vi "roboRIO v1.0 Enable Encoder.vi"(8 "error in (no error)":errorcluster, 9 "Enable":bool, 10 "Channel":T1, 11 "myRIO Ref In":T2) -> (0 "error out":errorcluster, 3 "myRIO Ref Out":T2)   [LabVIEW 2021]
uses:
  <vilib>/myRIO/Common/Instrument Driver Framework/Utilities/typedefs/myRIO v1.0 Reference.ctl
  <vilib>/myRIO/Common/Instrument Driver Framework/Utilities/typedefs/Generic FPGA Reference.ctl
  <vilib>/myRIO/Common/Instrument Driver Framework/myRIO v1.0/Encoder/typedefs/Encoder Channels Enum.ctl
  <vilib>/myRIO/Common/Instrument Driver Framework/roboRIO v1.0/Encoder/typedefs/roboRIO Encoder Channels FPGA Reference.ctl
  <vilib>/rvi/errors/niLvFpgaAdjustHostInterfaceError.vi
  <vilib>/rvi/interface/nirviReadWriteControl/nirviReadWriteControl.xnode
  <vilib>/rvi/interface/Simulation/niFpgaSimulationCallBeginRW.vi
  NiFpgaLv.dll
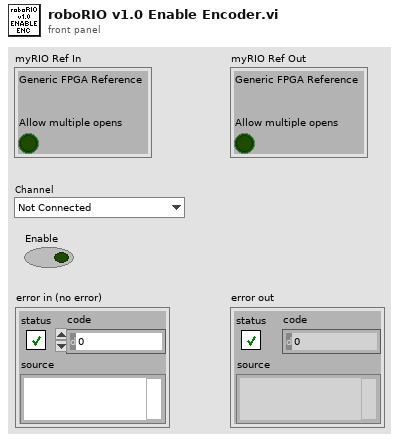
[diagram p1: front panel]
types:
  T1 = typedef "Encoder Channels Enum.ctl" = enum16{"Not Connected", "C/ENC0", "C/ENC1", "A/ENC", "A/ENC0", "A/ENC1", "A/ENC2", "A/ENC3", "A/ENC4", "A/ENC5", "A/ENC6", "A/ENC7", "A/ENC8", "A/ENC9", "B/ENC", "B/ENC0", "B/ENC1", "B/ENC2", "B/ENC3", "B/ENC4", "B/ENC5", "B/ENC6", "B/ENC7", "B/ENC8", "B/ENC9", "DIO/ENC0", "DIO/ENC1", "DIO/ENC2", "DIO/ENC3", "DIO/ENC4"}
  T2 = typedef "myRIO v1.0 Reference.ctl" = cluster{"Generic FPGA Reference":T3, "Allow multiple opens":bool}
  T3 = typedef "Generic FPGA Reference.ctl" = refnum<k20>
  T4 = typedef "roboRIO Encoder Channels FPGA Reference.ctl" = refnum<k20>
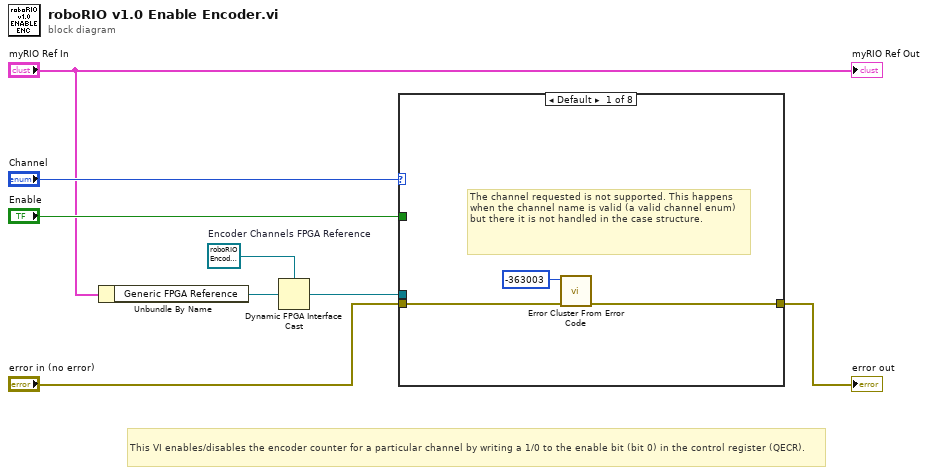
[diagram p0: block diagram]
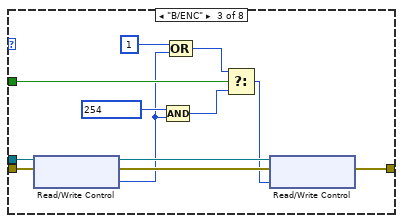
[diagram p3: hidden frame]
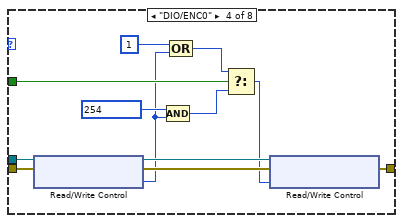
[diagram p4: hidden frame]
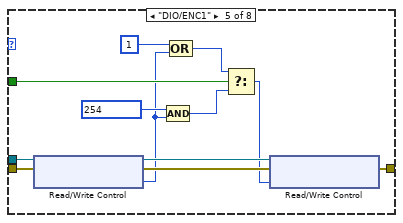
[diagram p5: hidden frame]
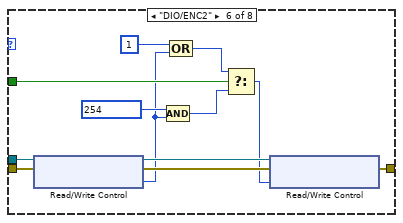
[diagram p6: hidden frame]
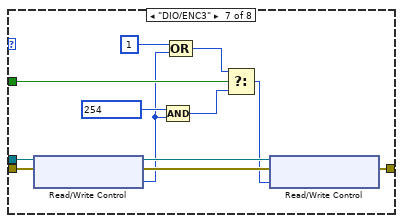
[diagram p7: hidden frame]
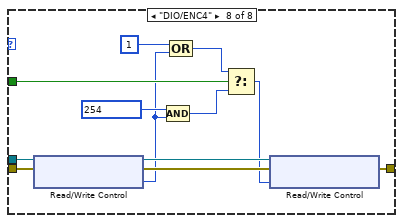
[diagram p8: hidden frame]
diagram:
  w8 = T4 refnum  # Encoder Channels FPGA Reference
  # "This VI enables/disables the encoder counter for a particular channel by writing a 1/0 to the enable bit (bit 0) in the control register (QECR)."
  n1 = Unbundle By Name("myRIO Ref In") -> ("Generic FPGA Reference"=w2:T3)
  n2 = Dynamic FPGA Interface Cast(Session In=w8, Type=w2) -> (Session Out=w7:T4)
  n3 = case shown="Default" "Channel" {
    tunnel: "error in (no error)" -> [w9 w12 w20 w32 w44 w56 w68 w80]
    tunnel: [w10 w12 w24 w36 w48 w60 w72 w84] -> w4
    tunnel: w7 -> [_ _ w21 w33 w45 w57 w69 w81]
    tunnel: "Enable" -> [_ _ w19 w31 w43 w55 w67 w79]
    frame Default {
      # "The channel requested is not supported. This happens when the channel name is valid (a valid channel enum) but there it is not handled in the case structure."
      n4 = call <vilib>:"Error Cluster From Error Code.vi"("error in (no error)"=w9, "error code (0)"=-363003) -> ("error out"=w10:errorcluster)  [unwired: 7 in]
    }
    frame "Not Connected" {
    }
    frame "B/ENC" {
      n5 = xnode "Read/Write Control"("FPGA VI Reference In"=w21, "error in"=w20) -> ("FPGA VI Reference Out"=w22:T4, "error out"=w23:errorcluster, "ENC.B.CNFG"=w15:u8)
      n6 = Compound Arithmetic op=AND(u8 254, w15) -> (w18:u8)
      n7 = Compound Arithmetic op=OR(u8 1, w15) -> (w14:u8)
      n8 = Select(t=w14, s=w19, f=w18) -> (s? t:f=w17:u8)
      n9 = xnode "Read/Write Control"("FPGA VI Reference In"=w22, "error in"=w23, "ENC.B.CNFG"=w17) -> ("error out"=w24:errorcluster)  [unwired: 1 out]
    }
    frame "DIO/ENC0" {
      n10 = xnode "Read/Write Control"("FPGA VI Reference In"=w33, "error in"=w32) -> ("FPGA VI Reference Out"=w34:T4, "error out"=w35:errorcluster, "ENC.DIO_0.CNFG"=w27:u8)
      n11 = Compound Arithmetic op=AND(u8 254, w27) -> (w30:u8)
      n12 = Compound Arithmetic op=OR(u8 1, w27) -> (w26:u8)
      n13 = Select(t=w26, s=w31, f=w30) -> (s? t:f=w29:u8)
      n14 = xnode "Read/Write Control"("FPGA VI Reference In"=w34, "error in"=w35, "ENC.DIO_0.CNFG"=w29) -> ("error out"=w36:errorcluster)  [unwired: 1 out]
    }
    frame "DIO/ENC1" {
      n15 = xnode "Read/Write Control"("FPGA VI Reference In"=w45, "error in"=w44) -> ("FPGA VI Reference Out"=w46:T4, "error out"=w47:errorcluster, "ENC.DIO_1.CNFG"=w39:u8)
      n16 = Compound Arithmetic op=AND(u8 254, w39) -> (w42:u8)
      n17 = Compound Arithmetic op=OR(u8 1, w39) -> (w38:u8)
      n18 = Select(t=w38, s=w43, f=w42) -> (s? t:f=w41:u8)
      n19 = xnode "Read/Write Control"("FPGA VI Reference In"=w46, "error in"=w47, "ENC.DIO_1.CNFG"=w41) -> ("error out"=w48:errorcluster)  [unwired: 1 out]
    }
    frame "DIO/ENC2" {
      n20 = xnode "Read/Write Control"("FPGA VI Reference In"=w57, "error in"=w56) -> ("FPGA VI Reference Out"=w58:T4, "error out"=w59:errorcluster, "ENC.DIO_2.CNFG"=w51:u8)
      n21 = Compound Arithmetic op=AND(u8 254, w51) -> (w54:u8)
      n22 = Compound Arithmetic op=OR(u8 1, w51) -> (w50:u8)
      n23 = Select(t=w50, s=w55, f=w54) -> (s? t:f=w53:u8)
      n24 = xnode "Read/Write Control"("FPGA VI Reference In"=w58, "error in"=w59, "ENC.DIO_2.CNFG"=w53) -> ("error out"=w60:errorcluster)  [unwired: 1 out]
    }
    frame "DIO/ENC3" {
      n25 = xnode "Read/Write Control"("FPGA VI Reference In"=w69, "error in"=w68) -> ("FPGA VI Reference Out"=w70:T4, "error out"=w71:errorcluster, "ENC.DIO_3.CNFG"=w63:u8)
      n26 = Compound Arithmetic op=AND(u8 254, w63) -> (w66:u8)
      n27 = Compound Arithmetic op=OR(u8 1, w63) -> (w62:u8)
      n28 = Select(t=w62, s=w67, f=w66) -> (s? t:f=w65:u8)
      n29 = xnode "Read/Write Control"("FPGA VI Reference In"=w70, "error in"=w71, "ENC.DIO_3.CNFG"=w65) -> ("error out"=w72:errorcluster)  [unwired: 1 out]
    }
    frame "DIO/ENC4" {
      n30 = xnode "Read/Write Control"("FPGA VI Reference In"=w81, "error in"=w80) -> ("FPGA VI Reference Out"=w82:T4, "error out"=w83:errorcluster, "ENC.DIO_4.CNFG"=w75:u8)
      n31 = Compound Arithmetic op=AND(u8 254, w75) -> (w78:u8)
      n32 = Compound Arithmetic op=OR(u8 1, w75) -> (w74:u8)
      n33 = Select(t=w74, s=w79, f=w78) -> (s? t:f=w77:u8)
      n34 = xnode "Read/Write Control"("FPGA VI Reference In"=w82, "error in"=w83, "ENC.DIO_4.CNFG"=w77) -> ("error out"=w84:errorcluster)  [unwired: 1 out]
    }
  }
  "error out" <- w4
  "myRIO Ref Out" <- "myRIO Ref In"
